vi "Command Dispatch.vi"(8 "error in (no error)":errorcluster, 10 "GUID-cmd-data":T1, 11 "Function in":refnum<class "Function.lvclass">) -> (0 "error out":errorcluster, 3 "Function out":refnum<class "Function.lvclass">)   [LabVIEW 2016, in "Function Actor.lvlib" / "Function.lvclass"]
uses:
  <userlib>/Common Components/Function Actor/Function.lvclass
  <userlib>/Common Components/Common/GUID-command-data.ctl
  <userlib>/Common Components/Common/Common.lvlib
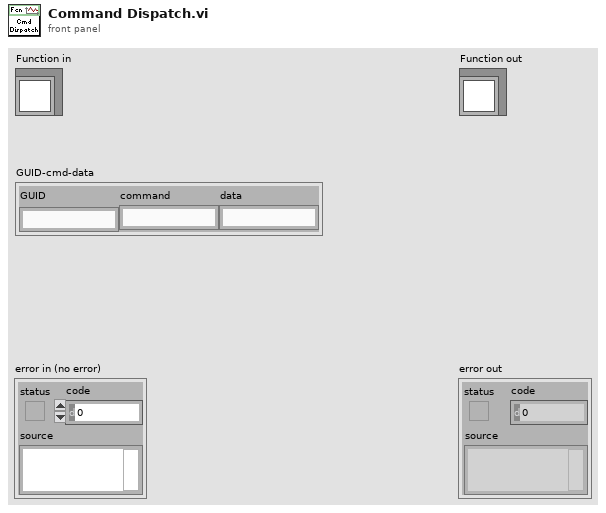
[diagram p1: front panel]
types:
  T1 = typedef "Common.lvlib/GUID-command-data.ctl" = cluster{"GUID":string, "command":string, "data":string}
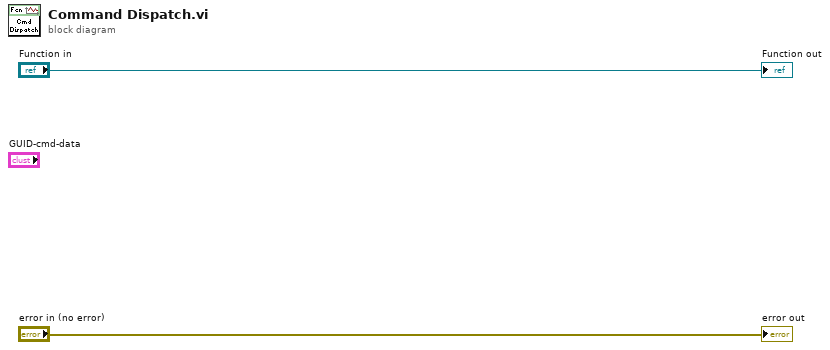
[diagram p0: block diagram]
diagram:
  "error out" <- "error in (no error)"
  "Function out" <- "Function in"
